vi "Log Manager.vi"(1 "Log_Manager_States":T2, 11 "Error IN":errorcluster, 12 "Station ID":T1) -> (4 "Log File OUT":path, 14 "Empty Path?":bool, 15 "Error OUT":errorcluster)   [LabVIEW 2011]
uses:
  Controls/Log_Manager_States.ctl
  Controls/Station ID.ctl
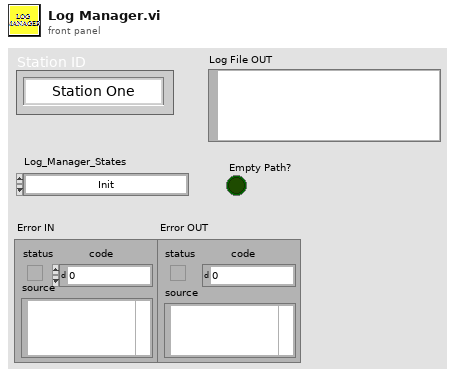
[diagram p1: front panel]
types:
  T1 = typedef "Station ID.ctl" = enum16{"Station One", "Station Two", "Station Three"}
  T2 = typedef "Log_Manager_States.ctl" = enum16{"Init", "Status", "Get Log File Path", "Log Data", "Write Header"}
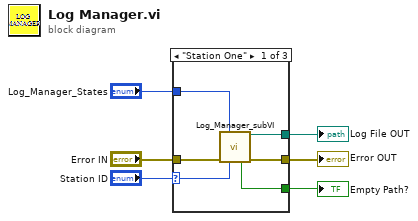
[diagram p0: block diagram]
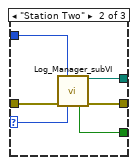
[diagram p2: hidden frame]
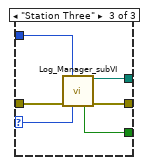
[diagram p3: hidden frame]
diagram:
  n1 = case shown="\"Station One\"" "Station ID" {
    selector: "Station ID" -> [w10 w16 w22]
    tunnel: "Log_Manager_States" -> [w9 w15 w21]
    tunnel: [w12 w18 w24] -> w5
    tunnel: "Error IN" -> [w11 w17 w23]
    tunnel: [w8 w14 w20] -> w2
    tunnel: [w7 w13 w19] -> w1
    frame "Station One" {
      n2 = call "Log_Manager_subVI.vi"("Log_Manager_States"=w9, "Error IN"=w11, "Station ID"=w10) -> ("Log File OUT"=w7:path, "Empty Path?"=w8:bool, "Error OUT"=w12:errorcluster)  [unwired: 10 in]
    }
    frame "Station Two" {
      n3 = call "Log_Manager_subVI.vi"("Log_Manager_States"=w15, "Error IN"=w17, "Station ID"=w16) -> ("Log File OUT"=w13:path, "Empty Path?"=w14:bool, "Error OUT"=w18:errorcluster)  [unwired: 10 in]
    }
    frame "Station Three" {
      n4 = call "Log_Manager_subVI.vi"("Log_Manager_States"=w21, "Error IN"=w23, "Station ID"=w22) -> ("Log File OUT"=w19:path, "Empty Path?"=w20:bool, "Error OUT"=w24:errorcluster)  [unwired: 10 in]
    }
  }
  "Error OUT" <- w5
  "Empty Path?" <- w2
  "Log File OUT" <- w1
